vi "room catch.vi"(8 "error in (no error)":errorcluster, 9 "Position in":T1) -> (0 "error out":errorcluster, 1 "Position out 2":T1)   [LabVIEW 2019]
uses:
  subVI/move/position cluster.ctl
  servo state.ctl
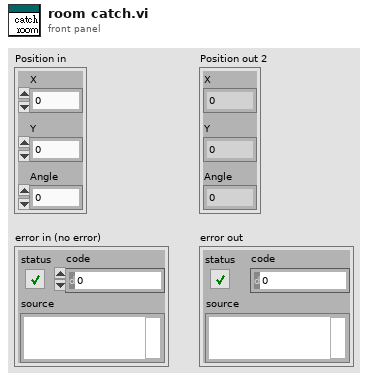
[diagram p1: front panel]
types:
  T1 = typedef "position cluster.ctl" = cluster{"X":dbl, "Y":dbl, "Angle":dbl}
  T2 = typedef "servo state.ctl" = enum16{"catch", "cam-1", "put", "side", "center", "side-2"}
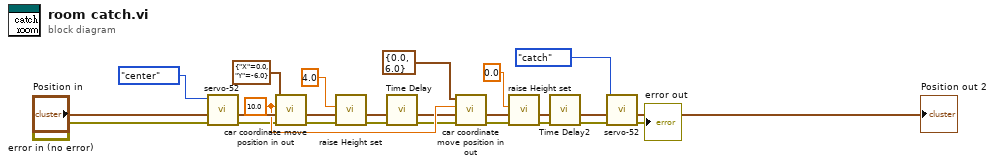
[diagram p0: block diagram]
diagram:
  w10 = 10.0 ("speed")
  n1 = call "servo-52.vi"("error in (no error)"="error in (no error)", "Enum"=servo_state."center") -> ("error out"=w3:errorcluster)  [unwired: 9 in]
  n2 = call "car coordinate move position in out.vi"("error in (no error)"=w3, "Position in"="Position in", "speed"=w10, "move"=cluster{"X":dbl, "Y":dbl} {"X"=0.0, "Y"=-6.0}) -> ("error out"=w5:errorcluster, "Position out"=w9:T1)  [unwired: 6 in]
  n3 = call "raise Height set.vi"("error in (no error)"=w5, "Height_cm"=4.0) -> ("error out"=w7:errorcluster)  [unwired: 9 in]
  n4 = call "Time Delay"("error in (no error)"=w7) -> ("error out"=w8:errorcluster)  [unwired: 10 in]
  n5 = call "car coordinate move position in out.vi"("error in (no error)"=w8, "Position in"=w9, "speed"=w10, "move"=cluster{"X":dbl, "Y":dbl} {"X"=0.0, "Y"=6.0}) -> ("error out"=w12:errorcluster, "Position out"=→"Position out 2":T1)  [unwired: 6 in]
  n6 = call "raise Height set.vi"("error in (no error)"=w12, "Height_cm"=0.0) -> ("error out"=w15:errorcluster)  [unwired: 9 in]
  n7 = call "Time Delay2"("error in (no error)"=w15) -> ("error out"=w16:errorcluster)  [unwired: 10 in]
  n8 = call "servo-52.vi"("error in (no error)"=w16, "Enum"=servo_state."catch") -> ("error out"=→"error out":errorcluster)  [unwired: 9 in]
